vi "Shooter calculations.vi.vi"() -> ()   [LabVIEW 2011]
panel:
  in  "stop":bool
  out "Speed":dbl
  in  "Basket Height (in)":dbl=98.0
  in  "Shooter Height (in)":dbl=50.0
  in  "Shooter Angle":dbl(slide)=55.0 scale=0.0..60.0
  in  "Range (ft)":dbl(slide)=20.0 scale=0.0..30.0
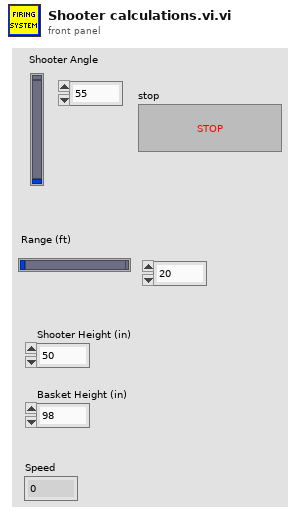
[diagram p1: front panel]
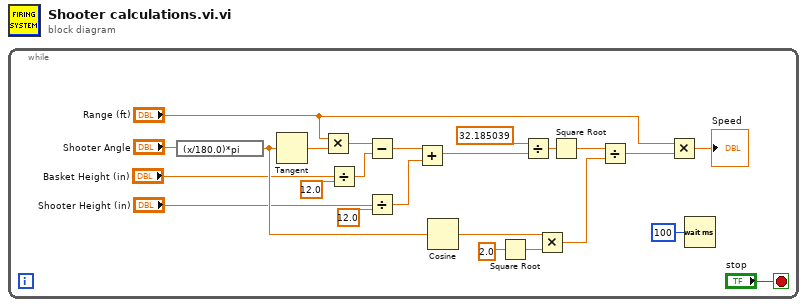
[diagram p0: block diagram]
diagram:
  n1 = while {
    stop <- "stop" stop-if-true
    n2 = expression code="(x/180.0)*pi"("Shooter Angle") -> (w9:dbl)
    n3 = Tangent(1:w9) -> (0:w21:dbl)
    n4 = Multiply(x="Range (ft)", y=w21) -> (x*y=w20:dbl)
    n5 = Divide(x="Basket Height (in)", y=12.0) -> (x/y=w4:dbl)
    n6 = Subtract(x=w20, y=w4) -> (x-y=w19:dbl)
    n7 = Divide(x="Shooter Height (in)", y=12.0) -> (x/y=w6:dbl)
    n8 = Add(x=w19, y=w6) -> (x+y=w17:dbl)
    n9 = Cosine(x=w9) -> (cos(x)=w22:dbl)
    n10 = Square Root(x=2.0) -> (sqrt(x)=w23:dbl)
    n11 = Divide(x=32.185039, y=w17) -> (x/y=w15:dbl)
    n12 = Multiply(x=w22, y=w23) -> (x*y=w18:dbl)
    n13 = Square Root(x=w15) -> (sqrt(x)=w14:dbl)
    n14 = Divide(x=w14, y=w18) -> (x/y=w13:dbl)
    n15 = Multiply(x="Range (ft)", y=w13) -> (x*y=→"Speed":dbl)
    n16 = Wait (ms)(milliseconds to wait=u32 100) -> ()  [unwired: 1 out]
  }
